vi "Shutdown.vi"(8 "error in (no error)":errorcluster, 11 "Managed Actor in":refnum<class "Managed Actor.lvclass">) -> (0 "error out":errorcluster, 3 "Managed Actor out":refnum<class "Managed Actor.lvclass">)   [LabVIEW 2023, in "Engine.lvlib" / "Managed Actor.lvlib" / "Managed Actor.lvclass"]
doc: "<b>Shutdown</b>\nThis routine is implemented in the stop actor override -> as a result, it is not necessary to call shutdown anywhere else, and any methods that need to be called prior to stop actor core can be implemented here.\n\n<b>Engine</b> - No methods implemented at the engine level\n\n<b>Managed Actor</b> This routine transmits a stop core to all subordinate actors"
uses:
  Library/Managed Actor.lvclass
  Library/Managed Actor.lvclass/Managed Actor.ctl
  Custom Controls/Subordinate.ctl
  builds/Framework/Actor Framework.lvlibp/1abvi3w/vi.lib/ActorFramework/Message Enqueuer/Message Enqueuer.lvclass
  Engine/Library/Engine.lvclass
  builds/Framework/Actor Framework.lvlibp/1abvi3w/vi.lib/ActorFramework/Stop Msg/Stop Msg.lvclass
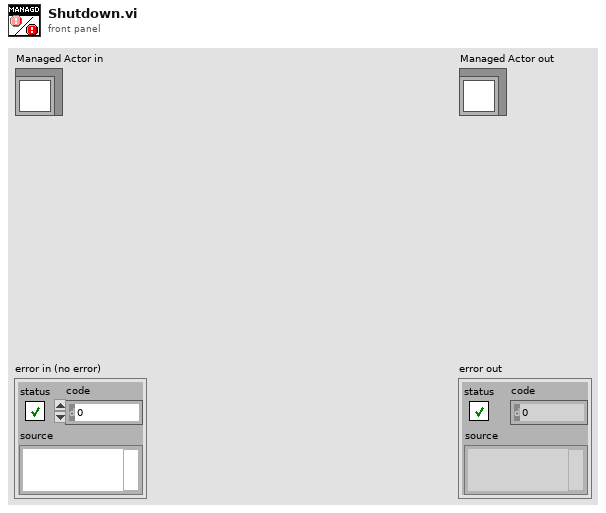
[diagram p1: front panel]
types:
  T1 = typedef "Engine.lvlib/Managed Actor.lvlib/Managed Actor.lvclass/Subordinate.ctl" = cluster{"Identifier":string, "Queue":refnum<class "Message Enqueuer.lvclass">, "PanelIndex":i32}
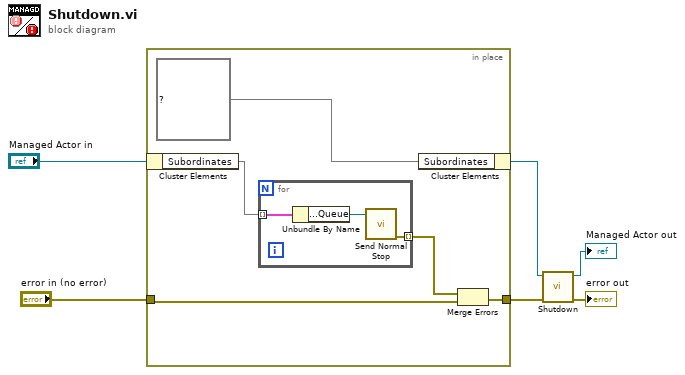
[diagram p0: block diagram]
diagram:
  n1 = in-place {
    in-place-border: "error in (no error)" -> [w9]
    in-place-border: [w8] -> w1
    n2 = in-place-cluster #1("Managed Actor in") -> ("Subordinates"=w10:map{string, T1})
    n3 = for {
      tunnel: w10 -> [w14] mode=indexing
      tunnel: [w12] -> w7 mode=indexing
      n4 = Unbundle By Name(w14) -> ("Subordinate.Queue"=w13:refnum<class "Message Enqueuer.lvclass">)
      n5 = call "Send Normal Stop.vi"("Message Enqueuer"=w13) -> ("error out"=w12:errorcluster)  [unwired: 10 in]
    }
    n6 = in-place-cluster #1("Subordinates"=map{string, T1} {}) -> (w3:refnum<class "Managed Actor.lvclass">)
    n7 = Merge Errors(w7, w9) -> (w8:errorcluster)
  }
  n8 = call-parent "Shutdown.vi"("error in (no error)"=w1, "Engine in"=w3) -> ("error out"=→"error out":errorcluster, "Engine out"=→"Managed Actor out":refnum<class "Managed Actor.lvclass">)  [unwired: 8 in]
